vi "CatFinder.vi"() -> ()   [LabVIEW 2014]
uses:
  <vilib>/Analysis/2dsp.llb/Real FFT.vi
  <vilib>/Analysis/2dsp.llb/Inverse Real FFT.vi
  <vilib>/Analysis/NI_AALPro.lvlib
panel:
  out "FFT":waveform(dbl)(graph)
  in  "do":i32
  in  "od":i32
  out "size(s)":i32
  out "After FFT":dbl[](graph)
  in  "FFT_b":bool
  in  "Length":dbl
  in  "Exit":bool
  in  "Play Sound":bool
  in  "Record":bool
  out "Signal":dynamicdata(graph)
  # "Pasmo czêstotliwoœci"
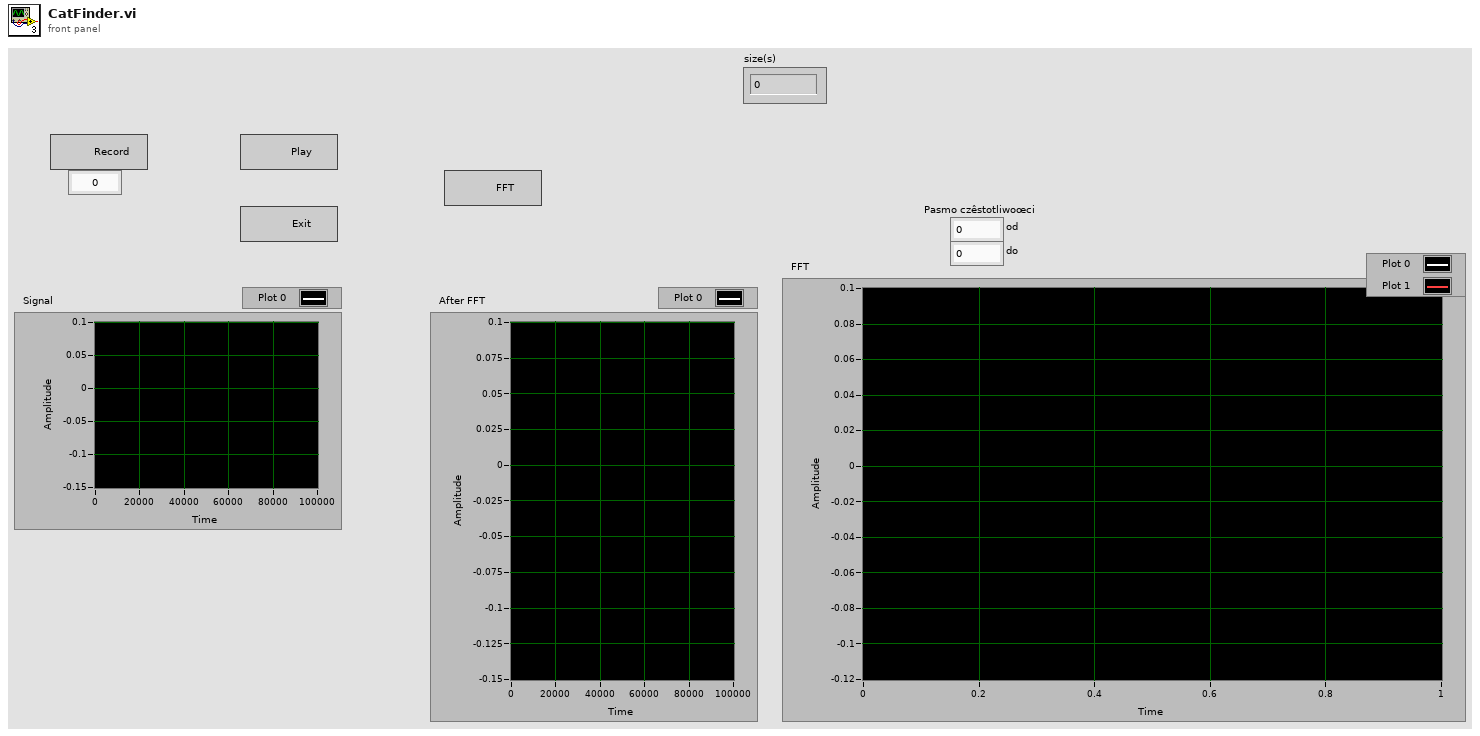
[diagram p1: front panel]
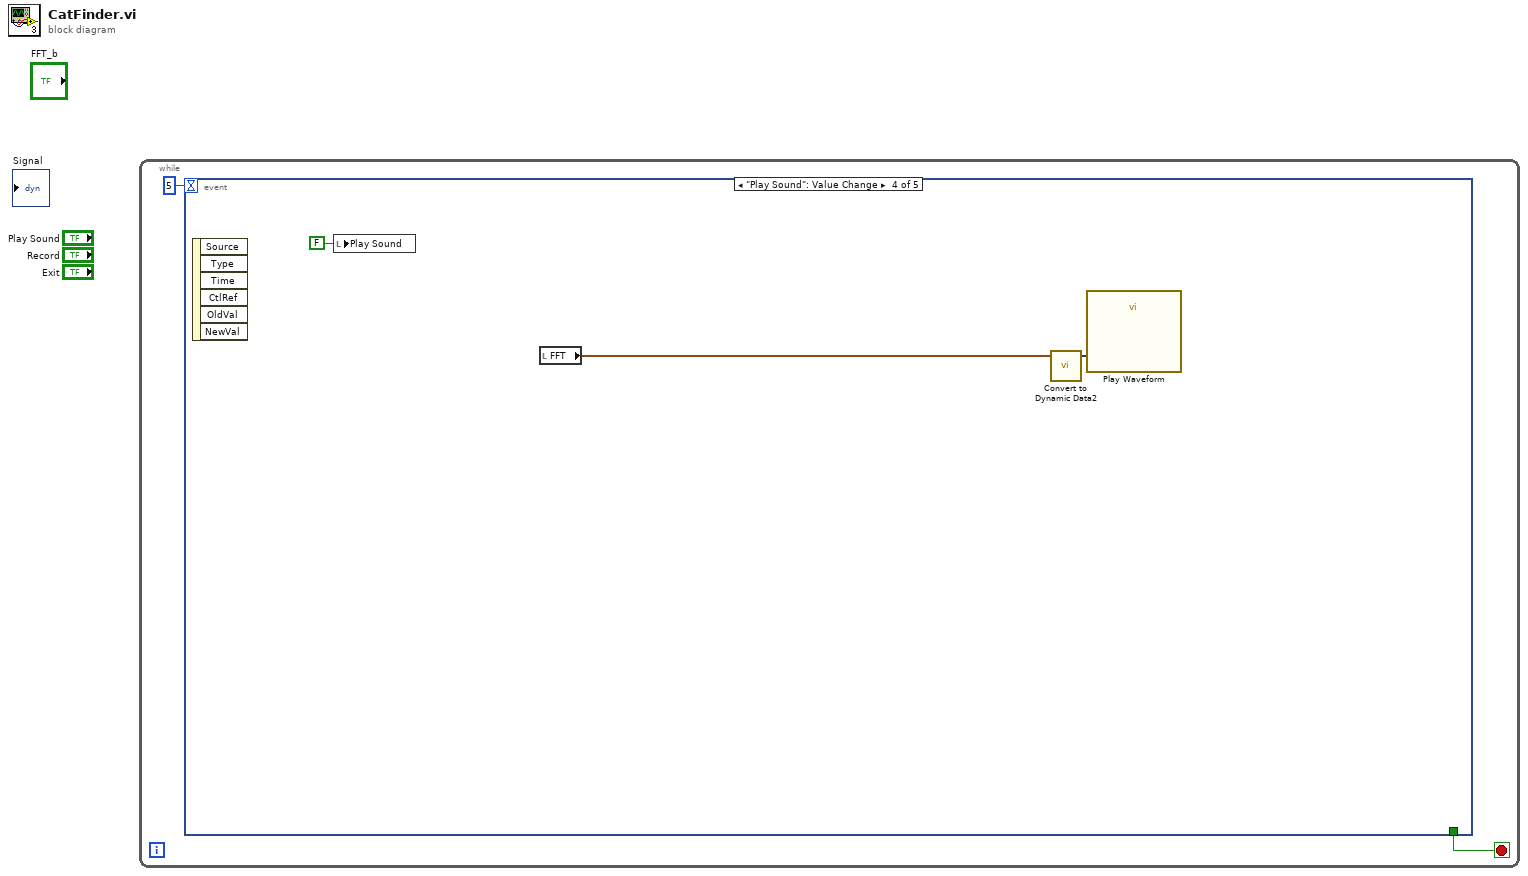
[diagram p0: block diagram]
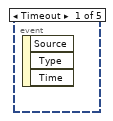
[diagram p2: hidden frame]
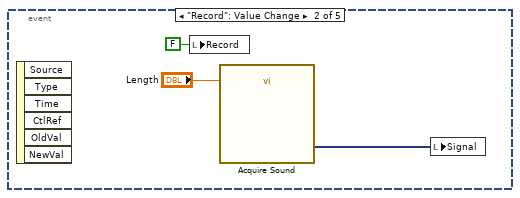
[diagram p3: hidden frame]
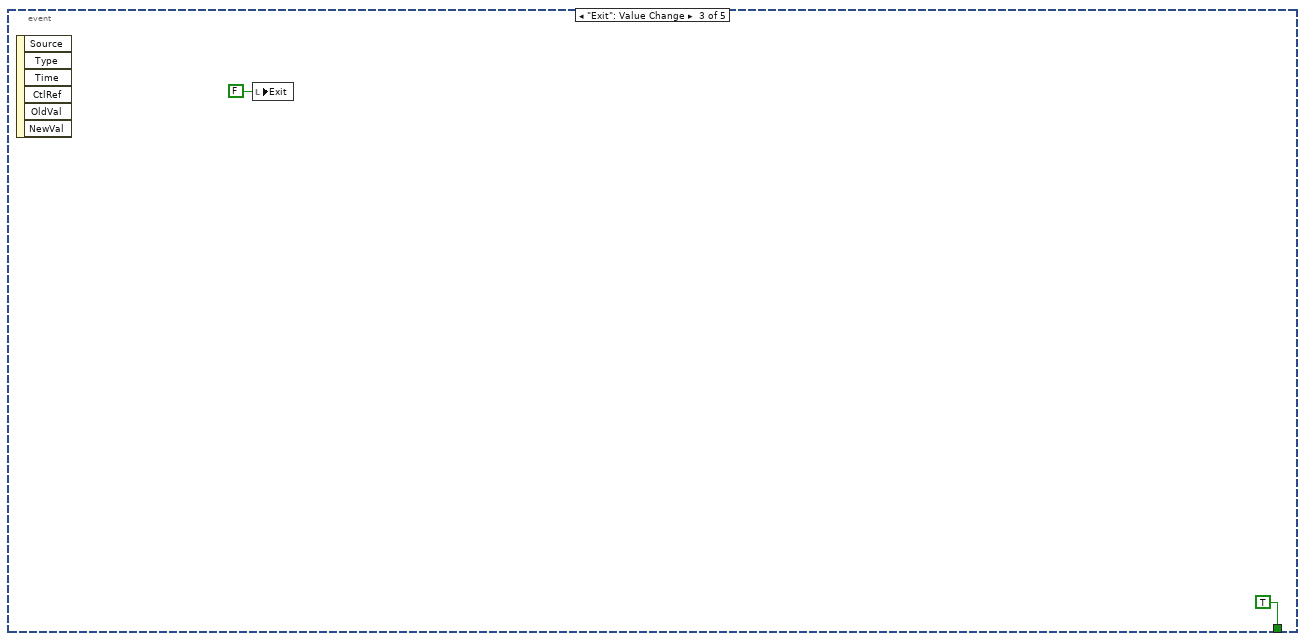
[diagram p4: hidden frame]
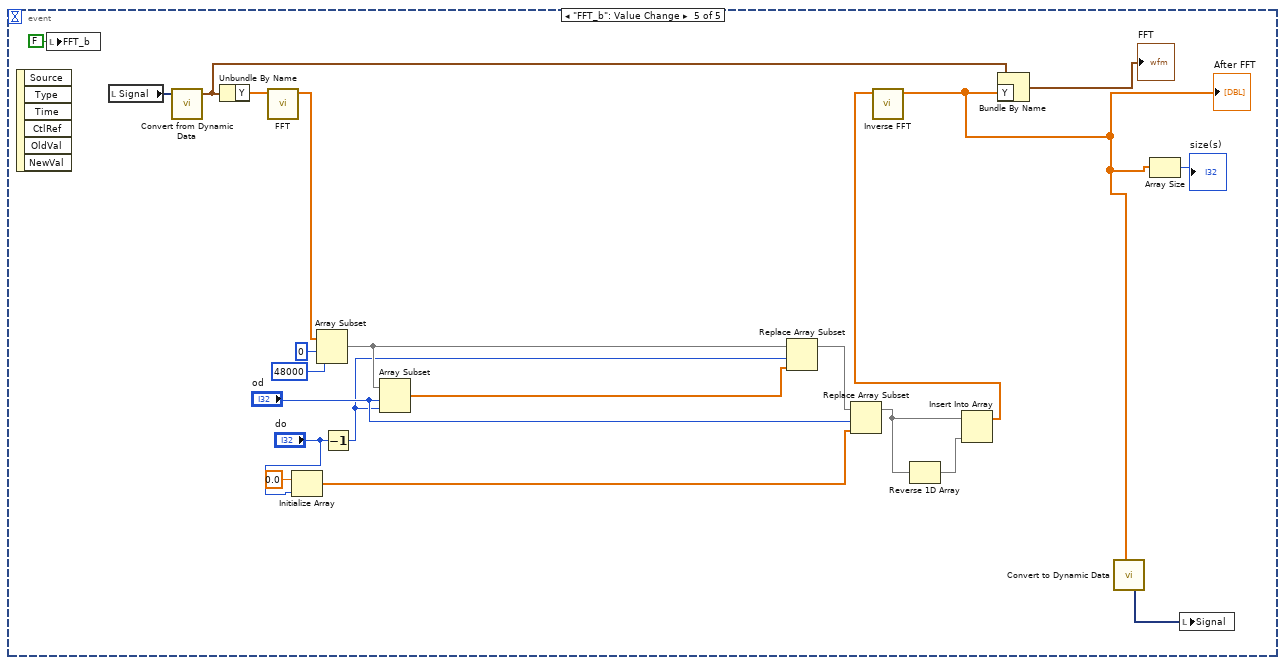
[diagram p5: hidden frame]
diagram:
  n1 = while {
    stop <- w1 stop-if-true
    n2 = event shown="[3] \"Play Sound\": Value Change" {
      selector: _ -> [_ _ _ _ _]
      dyn-events: _ -> [_ _ _ _ _]
      timeout: 5 -> [_ _ _ _ _]
      tunnel: [_ _ TRUE _ _] -> w1
      event Timeout {
        n3 = event-data() -> ()  [unwired: 1 in, 3 out]
      }
      event "Record": Value Change {
        n4 = event-data() -> ()  [unwired: 1 in, 6 out]
        n5 = local write "Record"(FALSE ("Record")) -> ()
        n6 = call "Acquire Sound"("Duration (s)"="Length") -> ("Data"=w3:dynamicdata)  [unwired: 17 in, 1 out]
        n7 = local write "Signal"(w3) -> ()
      }
      event "Exit": Value Change {
        n8 = event-data() -> ()  [unwired: 1 in, 6 out]
        n9 = local write "Exit"(FALSE ("Exit")) -> ()
      }
      event "Play Sound": Value Change {
        n10 = event-data() -> ()  [unwired: 1 in, 6 out]
        n11 = local write "Play Sound"(FALSE ("Play Sound")) -> ()
        n12 = local read "FFT"() -> (w8:waveform(dbl))
        n13 = call "Convert to Dynamic Data2"("Waveform"=w8) -> ("Dynamic Data Type"=w9:dynamicdata)  [unwired: 3 in]
        n14 = call "Play Waveform"("Data"=w9) -> ()  [unwired: 18 in, 1 out]
      }
      event "FFT_b": Value Change {
        n15 = event-data() -> ()  [unwired: 1 in, 6 out]
        n16 = local write "FFT_b"(FALSE ("FFT")) -> ()
        n17 = local read "Signal"() -> (w31:dynamicdata)
        n18 = call "Convert from Dynamic Data"("Dynamic Data Type"=w31) -> ("Waveform"=w14:waveform(dbl))  [unwired: 3 in]
        n19 = Unbundle By Name(w14) -> ("Y"=w15:dbl[])
        n20 = call-poly <vilib>:"FFT.vi"("X"=w15) -> ("FFT {X}"=w16:cdb[])  [unwired: 9 in, 1 out]
        n21 = Initialize Array(0.0 ("element"), "do") -> (w25:dbl[])
        n22 = Array Subset(array=w16, index=0, length=48000) -> (w28:cdb[])
        n23 = Decrement(x="do") -> (x-1=w17:i32)
        n24 = Array Subset(array=w28, index="od", length=w17) -> (w27:cdb[])
        n25 = Replace Array Subset(array=w28, new element=w27, index=w17) -> (w24:cdb[])
        n26 = Replace Array Subset(array=w24, new element=w25, index="od") -> (w23:cdb[])
        n27 = Reverse 1D Array(array=w23) -> (reversed array=w22:cdb[])
        n28 = Insert Into Array(array=w23, new element=w22) -> (w11:cdb[])  [unwired: 1 in]
        n29 = call-poly <vilib>:"Inverse FFT.vi"("FFT {X}"=w11) -> ("X"=w12:dbl[])  [unwired: 9 in, 1 out]
        "After FFT" <- w12
        n30 = Bundle By Name(cluster=w14, "Y"=w12) -> (→"FFT":waveform(dbl))
        n31 = call "Convert to Dynamic Data"("Array"=w12) -> ("Dynamic Data Type"=w20:dynamicdata)  [unwired: 3 in]
        n32 = Array Size(array=w12) -> (size(s)=→"size(s)":i32)
        n33 = local write "Signal"(w20) -> ()
      }
    }
  }
